vi "1DStandardConteniousPlot -Logging.vi"() -> ()   [LabVIEW 2024]
uses:
  <vilib>/DAQmx/read.llb/DAQmx Read (Analog Wfm 1Chan NSamp).vi
  <vilib>/DAQmx/create/channels.llb/DAQmx Create Channel (AI-Voltage-Basic).vi
  <vilib>/DAQmx/configure/timing.llb/DAQmx Timing (Sample Clock).vi
  <vilib>/DAQmx/miscellaneous.llb/DAQmx Fill In Error Info.vi
panel:
  out "Waveform Graph":waveform(dbl)(graph)
  in  "stop":bool
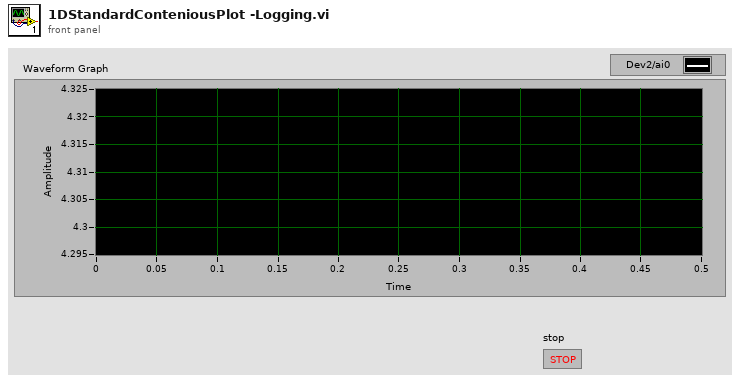
[diagram p1: front panel]
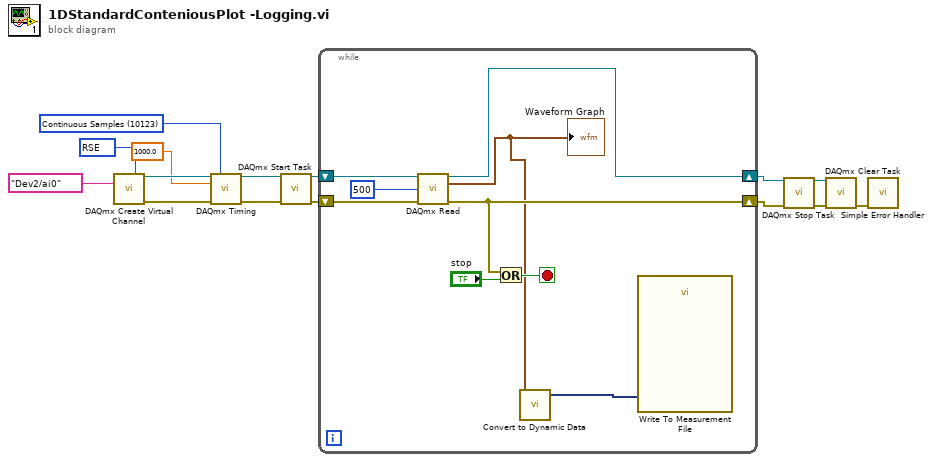
[diagram p0: block diagram]
diagram:
  w1 = 10083 items=["Default"=-1, "RSE"=10083, "NRSE"=10078, "Differential"=10106, "Pseudodifferential"=12529] ("input terminal configuration")
  w11 = 10123 items=["Finite Samples"=10178, "Continuous Samples"=10123, "Hardware Timed Single Point"=12522] ("sample mode")
  n1 = call-poly <vilib>:"DAQmx Create Virtual Channel.vi"("input terminal configuration"=w1, "physical channels"=tag "Dev2/ai0") -> ("task out"=w14:refnum<k21>, "error out"=w13:errorcluster)  [unwired: 12 in]
  n2 = call-poly <vilib>:"DAQmx Timing.vi"("task/channels in"=w14, "sample mode"=w11, "rate"=1000.0, "error in"=w13) -> ("task out"=w10:refnum<k21>, "error out"=w9:errorcluster)  [unwired: 10 in]
  n3 = call <vilib>:"DAQmx Start Task.vi"("task/channels in"=w10, "error in"=w9) -> ("task out"=w8:refnum<k21>, "error out"=w7:errorcluster)  [unwired: 12 in]
  n4 = while {
    shift-right: [w21] -> w6
    shift-left: w8 -> [w24]
    shift-right: [w19] -> w5
    shift-left: w7 -> [w23]
    stop <- w18 stop-if-true
    n5 = call-poly <vilib>:"DAQmx Read.vi"("task/channels in"=w24, "number of samples per channel"=500, "error in"=w23) -> ("task out"=w21:refnum<k21>, "data"=w17:waveform(dbl), "error out"=w19:errorcluster)  [unwired: 10 in]
    "Waveform Graph" <- w17
    n6 = Or(x=w19, y="stop") -> (x .or. y?=w18:bool)
    n7 = call "Convert to Dynamic Data"("Waveform"=w17) -> ("Dynamic Data Type"=w16:dynamicdata)  [unwired: 3 in]
    n8 = call "Write To Measurement File"("Signals"=w16) -> ()  [unwired: 16 in, 3 out]
  }
  n9 = call <vilib>:"DAQmx Stop Task.vi"("task/channels in"=w6, "error in"=w5) -> ("task out"=w4:refnum<k21>, "error out"=w3:errorcluster)  [unwired: 12 in]
  n10 = call <vilib>:"DAQmx Clear Task.vi"("task in"=w4, "error in"=w3) -> ("error out"=w2:errorcluster)  [unwired: 13 in]
  n11 = call <vilib>:"Simple Error Handler.vi"("error in (no error)"=w2) -> ()  [unwired: 4 in, 5 out]
